vi "Send TX Message.vi"(8 "error in (no error)":errorcluster, 10 "element":string, 11 "RxTx in":refnum<class "RxTx.lvclass">) -> (0 "error out":errorcluster, 3 "RxTx out":refnum<class "RxTx.lvclass">)   [LabVIEW 2018, in "RxTx.lvclass"]
uses:
  RxTx.lvclass
  RxTx.lvclass/RxTx.ctl
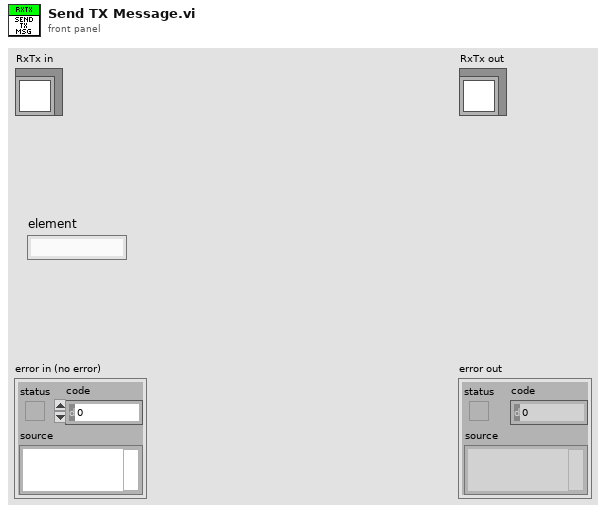
[diagram p1: front panel]
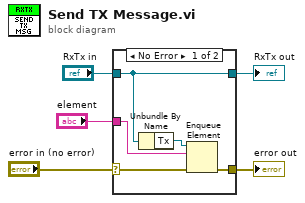
[diagram p0: block diagram]
diagram:
  n1 = case shown="No Error" "error in (no error)" {
    selector: "error in (no error)" -> [w8 w12]
    tunnel: [w7 w12] -> w4
    tunnel: [w10 w11] -> w2
    tunnel: "RxTx in" -> [w10 w11]
    tunnel: "element" -> [w6 _]
    frame No Error {
      n2 = Unbundle By Name(w10) -> ("Tx"=w9:refnum<queue>)
      n3 = Enqueue Element(queue=w9, element=w6, error in (no error)=w8) -> (error out=w7:errorcluster)  [unwired: 1 in, 2 out]
    }
    frame Error {
    }
  }
  "error out" <- w4
  "RxTx out" <- w2
